vi "Flat.vi"() -> ()   [LabVIEW 2020]
uses:
  <instrlib>/niDCPower/nidcpower.llb/niDCPower Output Function.ctl
  <instrlib>/niDCPower/nidcpower.llb/niDCPower Wait For Event - Event.ctl
  <instrlib>/niDCPower/nidcpower.llb/niDCPower Source Mode.ctl
  <vilib>/Analysis/baseanly.llb/Mean (DBL).vi
  <vilib>/Analysis/NI_AALBase.lvlib
panel:
  in  "voltage level":dbl[](array[numeric])=[4.0, 4.5, 5.0, 5.5, 6.0]
  out "load Voltage 3":dbl[](array[numeric]) format="%0.2f"
  out "load Current 3":dbl[](array[numeric]) format="%.5f"
  out "Vin Current 2":dbl[](array[numeric]) format="%.5f"
  out "Vin Voltage 2":dbl[](array[numeric]) format="%0.2f"
  out "Voltage":dbl format="%0.2f"
  out "Current":dbl format="%.5f"
  in  "error in (no error)":errorcluster
  in  "current level (A)":dbl=-0.005 format="%#_13g"
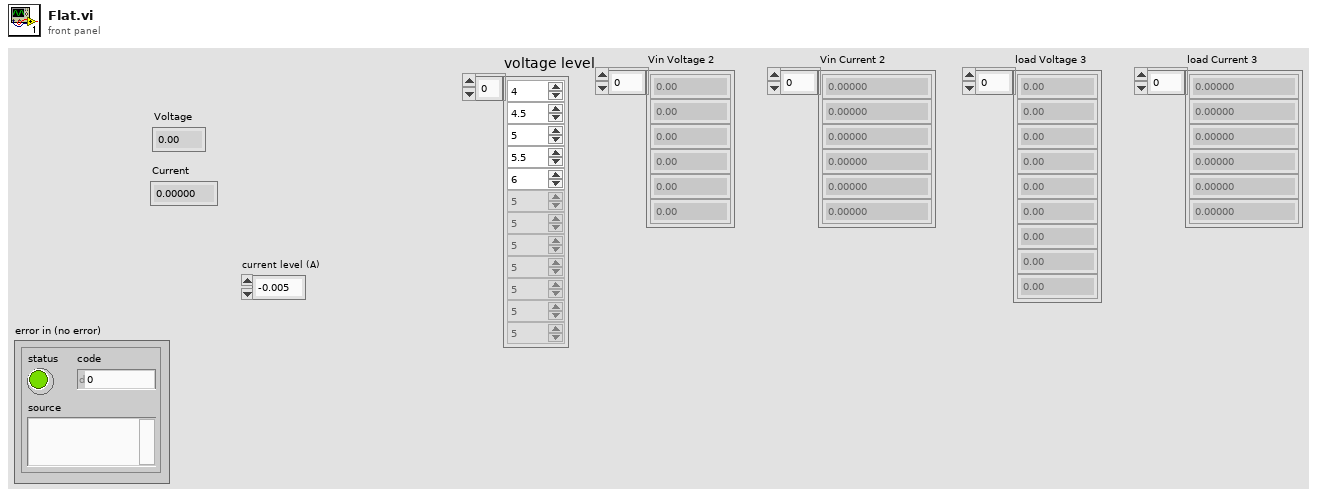
[diagram p1: front panel]
types:
  T1 = typedef "niDCPower Output Function.ctl" = i32
  T2 = typedef "niDCPower Source Mode.ctl" = i32
  T3 = typedef "niDCPower Wait For Event - Event.ctl" = i32
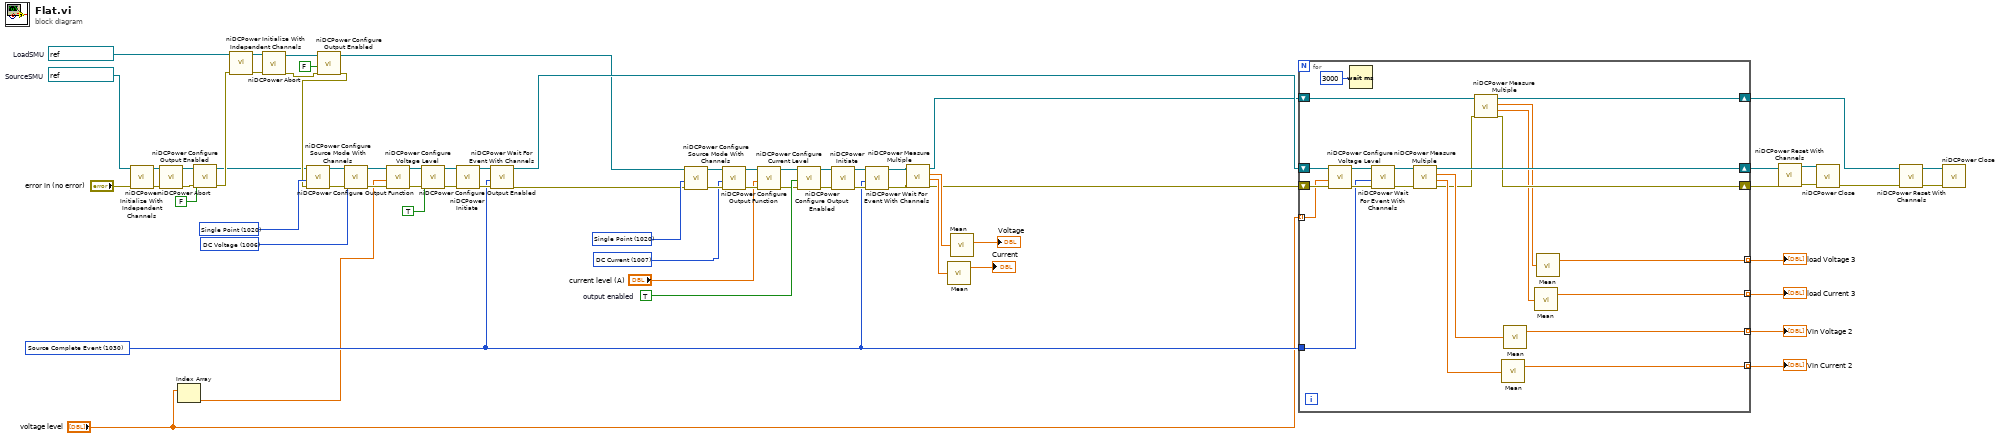
[diagram p0: block diagram]
diagram:
  w26 = T1 1006 items=["DC Voltage"=1006, "DC Current"=1007, "Pulse Voltage"=1049, "Pulse Current"=1050] ("output function")
  w19 = refnum<k15> "PXI1Slot8/0"  # SourceSMU
  w29 = T2 1020 items=["Single Point"=1020, "Sequence"=1021] ("source mode")
  w55 = refnum<k15> "PXI1Slot9/0"  # LoadSMU
  w23 = T3 1030 items=["Source Complete Event"=1030, "Measure Complete Event"=1031, "Sequence Iteration Complete Event"=1032, "Sequence Engine Done Event"=1033, "Pulse Complete Event"=1051, "Ready For Pulse Trigger Event"=1052] ("event")
  w68 = TRUE  # output enabled
  w44 = T1 1007 items=["DC Voltage"=1006, "DC Current"=1007, "Pulse Voltage"=1049, "Pulse Current"=1050] ("output function")
  w69 = T2 1020 items=["Single Point"=1020, "Sequence"=1021] ("source mode")
  n1 = call <instrlib>:"niDCPower Initialize With Independent Channels.vi"("error in (no error)"="error in (no error)", "resource name"=w19) -> ("error out"=w27:errorcluster, "instrument handle out"=w25:refnum<k15>)  [unwired: 8 in]
  n2 = call <instrlib>:"niDCPower Abort.vi"("error in (no error)"=w27, "instrument handle"=w25) -> ("error out"=w13:errorcluster, "instrument handle out"=w12:refnum<k15>)  [unwired: 8 in]
  n3 = Index Array(array="voltage level") -> (element=w1:dbl)  [unwired: 1 in]
  n4 = call <instrlib>:"niDCPower Configure Output Enabled.vi"("error in (no error)"=w13, "output enabled"=FALSE, "instrument handle"=w12) -> ("error out"=w7:errorcluster, "instrument handle out"=w5:refnum<k15>)  [unwired: 7 in]
  n5 = call <instrlib>:"niDCPower Initialize With Independent Channels.vi"("error in (no error)"=w7, "resource name"=w55) -> ("error out"=w56:errorcluster, "instrument handle out"=w57:refnum<k15>)  [unwired: 8 in]
  n6 = call <instrlib>:"niDCPower Abort.vi"("error in (no error)"=w56, "instrument handle"=w57) -> ("error out"=w9:errorcluster, "instrument handle out"=w8:refnum<k15>)  [unwired: 8 in]
  n7 = call <instrlib>:"niDCPower Configure Output Enabled.vi"("error in (no error)"=w9, "output enabled"=FALSE, "instrument handle"=w8) -> ("error out"=w6:errorcluster, "instrument handle out"=w4:refnum<k15>)  [unwired: 7 in]
  n8 = call <instrlib>:"niDCPower Configure Source Mode With Channels.vi"("error in (no error)"=w6, "source mode"=w29, "instrument handle"=w5) -> ("error out"=w34:errorcluster, "instrument handle out"=w35:refnum<k15>)  [unwired: 7 in]
  n9 = call <instrlib>:"niDCPower Configure Output Function.vi"("error in (no error)"=w34, "output function"=w26, "instrument handle"=w35) -> ("error out"=w36:errorcluster, "instrument handle out"=w38:refnum<k15>)  [unwired: 7 in]
  n10 = call <instrlib>:"niDCPower Configure Voltage Level.vi"("error in (no error)"=w36, "voltage level"=w1, "instrument handle"=w38) -> ("error out"=w37:errorcluster, "instrument handle out"=w39:refnum<k15>)  [unwired: 7 in]
  n11 = call <instrlib>:"niDCPower Configure Output Enabled.vi"("error in (no error)"=w37, "output enabled"=TRUE, "instrument handle"=w39) -> ("error out"=w30:errorcluster, "instrument handle out"=w31:refnum<k15>)  [unwired: 7 in]
  n12 = call <instrlib>:"niDCPower Initiate.vi"("error in (no error)"=w30, "instrument handle"=w31) -> ("error out"=w33:errorcluster, "instrument handle out"=w32:refnum<k15>)  [unwired: 8 in]
  n13 = call <instrlib>:"niDCPower Wait For Event With Channels.vi"("error in (no error)"=w33, "event"=w23, "instrument handle"=w32) -> ("error out"=w3:errorcluster, "instrument handle out"=w18:refnum<k15>)  [unwired: 7 in]
  n14 = call <instrlib>:"niDCPower Configure Source Mode With Channels.vi"("error in (no error)"=w3, "source mode"=w69, "instrument handle"=w4) -> ("error out"=w63:errorcluster, "instrument handle out"=w62:refnum<k15>)  [unwired: 7 in]
  n15 = call <instrlib>:"niDCPower Configure Output Function.vi"("error in (no error)"=w63, "output function"=w44, "instrument handle"=w62) -> ("error out"=w61:errorcluster, "instrument handle out"=w60:refnum<k15>)  [unwired: 7 in]
  n16 = call <instrlib>:"niDCPower Configure Current Level.vi"("error in (no error)"=w61, "current level"="current level (A)", "instrument handle"=w60) -> ("error out"=w59:errorcluster, "instrument handle out"=w58:refnum<k15>)  [unwired: 7 in]
  n17 = call <instrlib>:"niDCPower Configure Output Enabled.vi"("error in (no error)"=w59, "output enabled"=w68, "instrument handle"=w58) -> ("error out"=w67:errorcluster, "instrument handle out"=w66:refnum<k15>)  [unwired: 7 in]
  n18 = call <instrlib>:"niDCPower Initiate.vi"("error in (no error)"=w67, "instrument handle"=w66) -> ("error out"=w64:errorcluster, "instrument handle out"=w65:refnum<k15>)  [unwired: 8 in]
  n19 = call <instrlib>:"niDCPower Wait For Event With Channels.vi"("error in (no error)"=w64, "event"=w23, "instrument handle"=w65) -> ("error out"=w53:errorcluster, "instrument handle out"=w54:refnum<k15>)  [unwired: 7 in]
  n20 = call <instrlib>:"niDCPower Measure Multiple.vi"("error in (no error)"=w53, "instrument handle"=w54) -> ("error out"=w46:errorcluster, "current measurements"=w50:dbl[], "voltage measurements"=w48:dbl[], "instrument handle out"=w17:refnum<k15>)  [unwired: 6 in]
  n21 = call-poly <vilib>:"Mean.vi"("X"=w50) -> ("mean"=→"Current":dbl)  [unwired: 1 out]
  n22 = call-poly <vilib>:"Mean.vi"("X"=w48) -> ("mean"=→"Voltage":dbl)  [unwired: 1 out]
  n23 = for {
    tunnel: "voltage level" -> [w82] mode=indexing
    tunnel: w23 -> [w81]
    shift-right: [w83] -> w45
    shift-left: w18 -> [w87]
    shift-right: [w75] -> w22
    shift-left: w46 -> [w85]
    tunnel: [w80] -> w21 mode=indexing
    tunnel: [w79] -> w20 mode=indexing
    shift-right: [w73] -> w14
    shift-left: w17 -> [w74]
    tunnel: [w77] -> w15 mode=indexing
    tunnel: [w78] -> w16 mode=indexing
    n24 = call <instrlib>:"niDCPower Configure Voltage Level.vi"("error in (no error)"=w85, "voltage level"=w82, "instrument handle"=w87) -> ("error out"=w86:errorcluster, "instrument handle out"=w88:refnum<k15>)  [unwired: 7 in]
    n25 = Wait (ms)(milliseconds to wait=u32 3000) -> ()  [unwired: 1 out]
    n26 = call <instrlib>:"niDCPower Wait For Event With Channels.vi"("error in (no error)"=w86, "event"=w81, "instrument handle"=w88) -> ("error out"=w90:errorcluster, "instrument handle out"=w89:refnum<k15>)  [unwired: 7 in]
    n27 = call <instrlib>:"niDCPower Measure Multiple.vi"("error in (no error)"=w90, "instrument handle"=w89) -> ("error out"=w76:errorcluster, "current measurements"=w91:dbl[], "voltage measurements"=w84:dbl[], "instrument handle out"=w83:refnum<k15>)  [unwired: 6 in]
    n28 = call <instrlib>:"niDCPower Measure Multiple.vi"("error in (no error)"=w76, "instrument handle"=w74) -> ("error out"=w75:errorcluster, "current measurements"=w71:dbl[], "voltage measurements"=w72:dbl[], "instrument handle out"=w73:refnum<k15>)  [unwired: 6 in]
    n29 = call-poly <vilib>:"Mean.vi"("X"=w91) -> ("mean"=w79:dbl)  [unwired: 1 out]
    n30 = call-poly <vilib>:"Mean.vi"("X"=w84) -> ("mean"=w80:dbl)  [unwired: 1 out]
    n31 = call-poly <vilib>:"Mean.vi"("X"=w71) -> ("mean"=w78:dbl)  [unwired: 1 out]
    n32 = call-poly <vilib>:"Mean.vi"("X"=w72) -> ("mean"=w77:dbl)  [unwired: 1 out]
  }
  "Vin Voltage 2" <- w21
  "Vin Current 2" <- w20
  "load Voltage 3" <- w15
  "load Current 3" <- w16
  n33 = call <instrlib>:"niDCPower Reset With Channels.vi"("error in (no error)"=w22, "instrument handle"=w45) -> ("error out"=w52:errorcluster, "instrument handle out"=w51:refnum<k15>)  [unwired: 8 in]
  n34 = call <instrlib>:"niDCPower Close.vi"("error in (no error)"=w52, "instrument handle"=w51) -> ("error out"=w42:errorcluster)  [unwired: 9 in]
  n35 = call <instrlib>:"niDCPower Reset With Channels.vi"("error in (no error)"=w42, "instrument handle"=w14) -> ("error out"=w41:errorcluster, "instrument handle out"=w40:refnum<k15>)  [unwired: 8 in]
  n36 = call <instrlib>:"niDCPower Close.vi"("error in (no error)"=w41, "instrument handle"=w40) -> ()  [unwired: 9 in, 1 out]
